vi "WPI_CameraBuild Camera IP Address.vi"(8 "Camera on switch? (T)":bool=TRUE, 11 "Robot Address":string) -> (3 "Camera Address":string)   [LabVIEW 2017]
doc: "This VI returns the IP addres of the camera based on how the camera is conencted to the cRIO. If connected to the second port of the 8-slot cRIO, it returns the traditional 192.168.0.90 address, otherwise it constructs the camera IP from the robot IP."
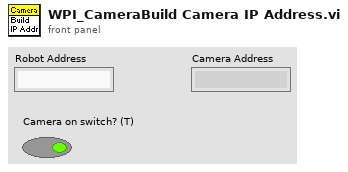
[diagram p1: front panel]
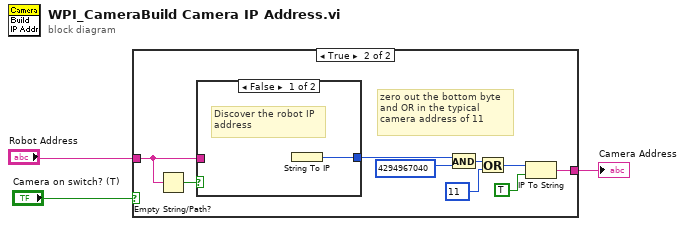
[diagram p0: block diagram]
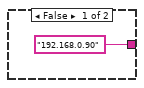
[diagram p2: hidden frame]
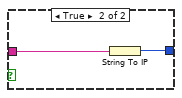
[diagram p3: hidden frame]
diagram:
  n1 = case shown="True" "Camera on switch? (T)" {
    tunnel: ["192.168.0.90" ("name") w8] -> w3
    tunnel: "Robot Address" -> [_ w6]
    frame False {
    }
    frame True {
      # "zero out the bottom byte\nand OR in the typical\ncamera address of 11"
      n2 = Empty String/Path?(string/path=w6) -> (empty?=w13:bool)
      n3 = case shown="False" w13 {
        tunnel: [w14 w16] -> w7
        tunnel: w6 -> [_ w15]
        frame False {
          # "Discover the robot IP\naddress"
          n4 = String To IP() -> (0:w14:u32)  [unwired: 1 in]
        }
        frame True {
          n5 = String To IP(1:w15) -> (0:w16:u32)
        }
      }
      n6 = And(x=w7, y=u32 4294967040) -> (x .and. y?=w12:u32)
      n7 = Or(x=w12, y=u32 11) -> (x .or. y?=w9:u32)
      n8 = IP To String(1:TRUE ("dot notation? (F)"), 2:w9) -> (0:w8:string)
    }
  }
  "Camera Address" <- w3
